vi "set_FPGA_wrapper.vi"(8 "error in (no error)":errorcluster, 10 "GenericFPGAWrapper.lvclass":refnum<class "GenericFPGAWrapper.lvclass">, 11 "TrajectoryMG100122GenericFPGA in":refnum<class "TrajectoryMG100122GenericFPGA.lvclass">) -> (0 "error out":errorcluster, 3 "TrajectoryMG100122GenericFPGA out":refnum<class "TrajectoryMG100122GenericFPGA.lvclass">)   [LabVIEW 2010, in "TrajectoryMG100122GenericFPGA.lvclass"]
uses:
  TrajectoryMG100122GenericFPGA.lvclass
  FPGAWrapper/GenericFPGAWrapper/GenericFPGAWrapper/GenericFPGAWrapper.lvclass
  TrajectoryMG100122GenericFPGA.lvclass/TrajectoryMG100122GenericFPGA.ctl
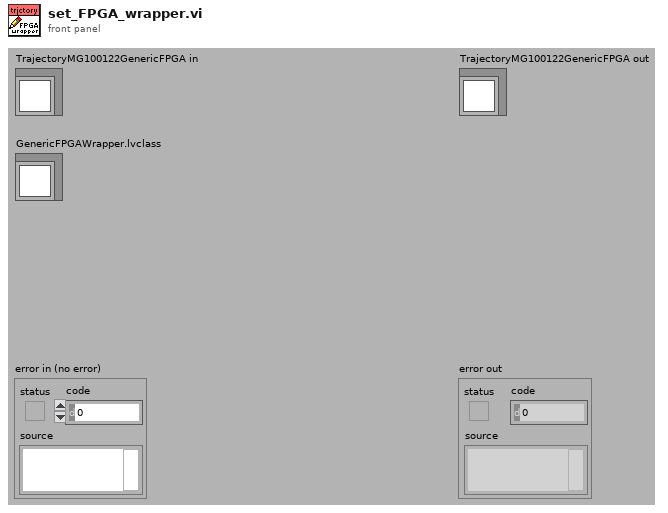
[diagram p1: front panel]
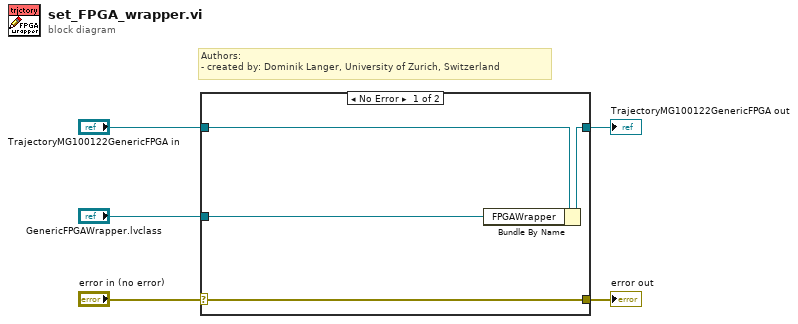
[diagram p0: block diagram]
diagram:
  # "Authors: \n- created by: Dominik Langer, University of Zurich, Switzerland"
  n1 = case shown="No Error" "error in (no error)" {
    selector: "error in (no error)" -> [w9 w10]
    tunnel: [w9 w10] -> w4
    tunnel: [w7 w11] -> w2
    tunnel: "TrajectoryMG100122GenericFPGA in" -> [w8 w11]
    tunnel: "GenericFPGAWrapper.lvclass" -> [w6 _]
    frame No Error {
      n2 = Bundle By Name(cluster=w8, "FPGAWrapper"=w6) -> (w7:refnum<class "TrajectoryMG100122GenericFPGA.lvclass">)
    }
    frame Error {
    }
  }
  "error out" <- w4
  "TrajectoryMG100122GenericFPGA out" <- w2
